vi "RSZVB Set Virtual Transform Balanced Circuit Model.vi"(6 "Logical Port Number (1)":i32=1, 7 "Circuit Model (5: Serial Cs, shunt L)":i32(ring)=5 items=["File import, no circuit model", "Serial Touchstone (.s2p) data, shunt L", "Serial Touchstone (.s2p) data, shunt C", "Shunt L, serial Touchstone (.s2p) data", "Shunt C, serial Touchstone (.s2p) data", "Serial Cs, shunt L", "Serial Ls, shunt C", "Serial Cs, shunt C", "Serial Ls, shunt L", "Shunt L, serial Cs", "Shunt C, serial Ls", "Shunt C, serial Cs", "Shunt L, serial Ls"], 8 "error in (no error)":errorcluster {"code" format="%.0x"}, 9 "Function Type (0: Deembedding)":i32(ring) items=["Deembedding", "Embedding"], 10 "Channel (1)":i32=1, 11 "VISA session":refnum<visa-resource-name>) -> (0 "error out":errorcluster {"code" format="%.0x"}, 3 "dup VISA session":refnum<visa-resource-name>)   [LabVIEW 2011]
doc: "This VI selects the circuit model for balanced port deembedding/embedding.\n\nRemote-control command(s):\nCALCulate<Ch>:TRANsform:VNETworks:BALanced:DEEMbedding<Log_pt>:TNDefinition\nFIMPort | STSL | STSC | SLST | SCST | CSSL | LSSC | CSSC | LSSL | SLCS | SCLS | SCCS | SLLS \n\nCALCulate<Ch>:TRANsform:VNETworks:BALanced:EMBedding<Log_pt>:TNDefinition\nFIMPort | STSL | STSC | SLST | SCST | CSSL | LSSC | CSSC | LSSL | SLCS | SCLS | SCCS | SLLS"
uses:
  _utility/RSZVB Global Data.vi
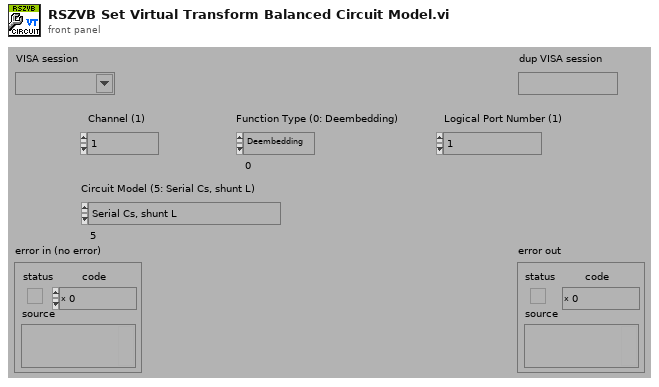
[diagram p1: front panel]
types:
  T1 = cluster{"Error Checking (T: On)":bool, "Installed Options":string[], "Data Valid?":bool, "Ports":i32, "Model":string[], "Option Checking (T: On)":bool}[]
  T2 = cluster{"Error Checking (T: On)":bool, "Installed Options":string[], "Data Valid?":bool, "Ports":i32, "Model":string[], "Option Checking (T: On)":bool}
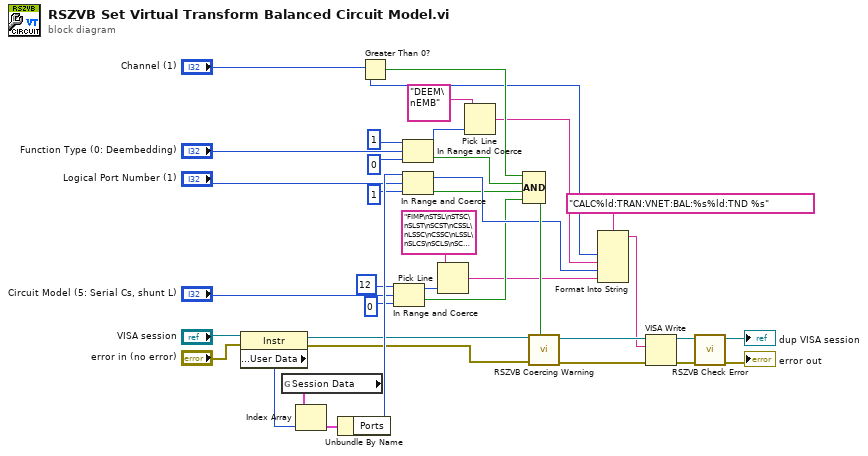
[diagram p0: block diagram]
diagram:
  n1 = property class="Instr"(reference="VISA session", error in="error in (no error)") -> (reference out=w26:refnum<visa-resource-name>, error out=w27:errorcluster, "General Settings:User Data"=w31:u32)
  n2 = global read "RSZVB Global Data.vi" "Session Data"() -> (w30:T1)
  n3 = Index Array(array=w30, index=w31) -> (element=w29:T2)
  n4 = Unbundle By Name(w29) -> ("Ports"=w28:i32)
  n5 = Greater Than 0?(x="Channel (1)") -> (x > 0?=w23:bool)
  n6 = In Range and Coerce(upper limit=12 ("lower limit"), x="Circuit Model (5: Serial Cs, shunt L)", lower limit=0) -> (coerced(x)=w4:i32, In Range?=w2:bool)
  n7 = In Range and Coerce(upper limit=1 ("lower limit"), x="Function Type (0: Deembedding)", lower limit=0) -> (coerced(x)=w17:i32, In Range?=w20:bool)
  n8 = In Range and Coerce(upper limit=w28, x="Logical Port Number (1)", lower limit=1) -> (coerced(x)=w19:i32, In Range?=w15:bool)
  n9 = Pick Line(multi-line string="FIMP\nSTSL\nSTSC\nSLST\nSCST\nCSSL\nLSSC\nCSSC\nLSSL\nSLCS\nSCLS\nSCCS\nSLLS", line index=w4) -> (output string=w1:string)  [unwired: 1 in]
  n10 = Pick Line(multi-line string="DEEM\nEMB", line index=w17) -> (output string=w16:string)  [unwired: 1 in]
  n11 = Compound Arithmetic op=AND(w23, w20, w15, w2) -> (w22:bool)
  n12 = call "RSZVB Coercing Warning.vi"("In Range?"=w22, "error in (no error)"=w27, "VISA session"=w26) -> ("error out"=w36:errorcluster, "dup VISA session"=w37:refnum<visa-resource-name>)  [unwired: 7 in]
  n13 = Format Into String(format string="CALC%ld:TRAN:VNET:BAL:%s%ld:TND %s", "Channel (1)", w16, w19, w1) -> (resulting string=w32:string)  [unwired: 2 in, 1 out]
  n14 = VISA Write(VISA resource name=w37, write buffer=w32, error in (no error)=w36) -> (VISA resource name out=w34:refnum<visa-resource-name>, error out=w35:errorcluster)  [unwired: 1 out]
  n15 = call "RSZVB Check Error.vi"("error in (no error)"=w35, "VISA session"=w34) -> ("error out"=→"error out":errorcluster, "dup VISA session"=→"dup VISA session":refnum<visa-resource-name>)  [unwired: 8 in]
